vi "KonverzeDat(SubVI).vi"(1 "Vstupni OpenSignals .txt export":dbl[][](array[numeric])) -> (0 "Data ve spravnem formatu":dbl[](array[numeric]))   [LabVIEW 2025]
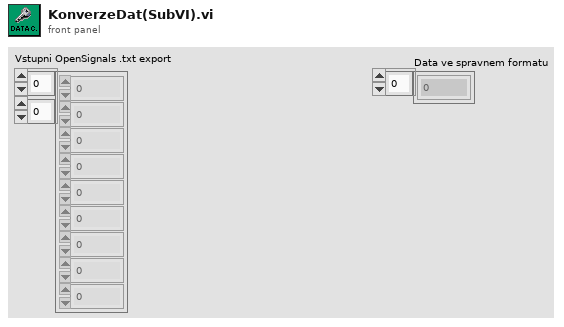
[diagram p1: front panel]
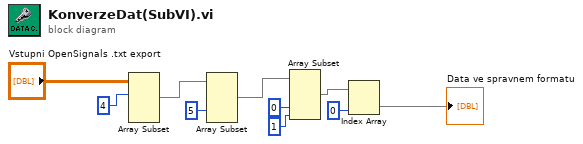
[diagram p0: block diagram]
diagram:
  n1 = Array Subset(array="Vstupni OpenSignals .txt export", index (row)=4 ("index")) -> (w3:dbl[][])  [unwired: 3 in]
  n2 = Array Subset(array=w3, index (col)=5 ("index")) -> (w6:dbl[][])  [unwired: 3 in]
  n3 = Array Subset(array=w6, index (col)=0 ("index"), length (col)=1 ("length")) -> (w8:dbl[][])  [unwired: 2 in]
  n4 = Index Array(array=w8, index (col)=0 ("disabled index (col)")) -> (element=→"Data ve spravnem formatu":dbl[])  [unwired: 1 in]
